vi "Unflatten Value.vi"(8 "Error In":errorcluster, 10 "Value":string, 11 "Flt Array In":refnum<class "1D Flt.lvclass">) -> (0 "Error Out":errorcluster, 3 "Flt Array Out":refnum<class "1D Flt.lvclass">)   [LabVIEW 2017, in "Tree API.lvlib" / "1D Flt.lvclass"]
uses:
  1D Flt.lvclass
  Tree Manager/Tree.lvclass
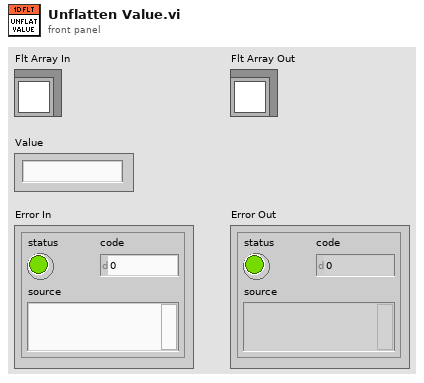
[diagram p1: front panel]
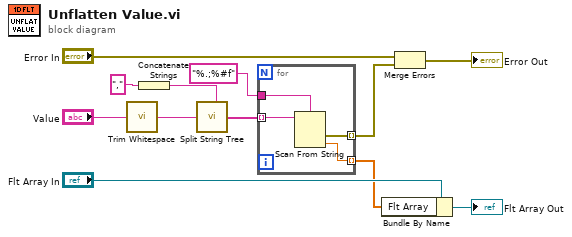
[diagram p0: block diagram]
diagram:
  n1 = call <vilib>:"Trim Whitespace.vi"("string"="Value") -> ("trimmed string"=w1:string)  [unwired: 1 in]
  n2 = Concatenate Strings("," ("Separator (,)")) -> (w2:string)
  n3 = call "Split String Tree.vi"("Split Pattern"=w2, "Input String"=w1) -> ("Split String"=w10:string[])  [unwired: 5 in]
  n4 = for {
    tunnel: w10 -> [w16] mode=indexing
    tunnel: [w15] -> w9 mode=indexing
    tunnel: [w14] -> w8 mode=indexing
    tunnel: "%.;%#f" ("initial string") -> [w13]
    n5 = Scan From String(format string=w13, input string=w16) -> (error out=w14:errorcluster, output 1=w15:dbl)  [unwired: 3 in, 2 out]
  }
  n6 = Bundle By Name(cluster="Flt Array In", "Flt Array"=w9) -> (→"Flt Array Out":refnum<class "1D Flt.lvclass">)
  n7 = Merge Errors("Error In", w8) -> (→"Error Out":errorcluster)
